vi "Time Profile Logger using LV2.vi"(6 "Command (Log)":T1=enum."Log", 7 "Log Path (Optional)":path, 8 "error in (no error)":errorcluster, 10 "Optional Tags":string[](array[string]), 11 "Primary Tag":string) -> (0 "error out":errorcluster, 2 "Profile Data[][]":string[][](array[string]), 3 "Log Path":path)   [LabVIEW 2016, in "SLL Debug.lvlib"]
doc: "Simple Time Profile Logger with multiple tag inputs. \n\n<b>Important!</b> -The final call to this VI needs to invoke \"Flush and Close\" command to log to file.\n\nDuring logging, the items are just put into a queue. Only during close operation, the data is parsed and logged to file. Supports logging into *.bin, *.csv & *.txt based on the file extension provided to the file name."
uses:
  SLL Debug.lvlib
  _Typedefs/Time Profile Logger Command.ctl
  <vilib>/Utility/file.llb/Write Delimited Spreadsheet (string).vi
  SLL String/SLL String.lvlib
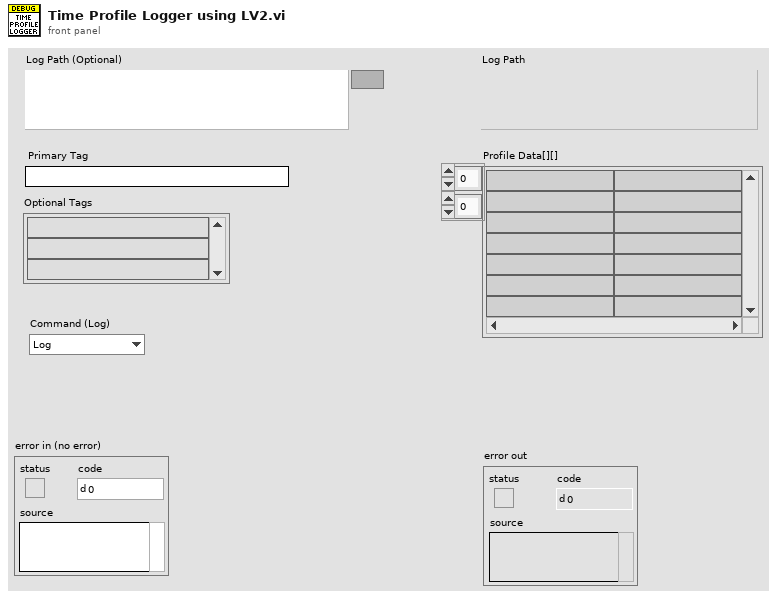
[diagram p1: front panel]
types:
  T1 = typedef "SLL Debug.lvlib/Time Profile Logger Command.ctl" = enum16{"Force Initialize", "Log", "Flush and Close"}
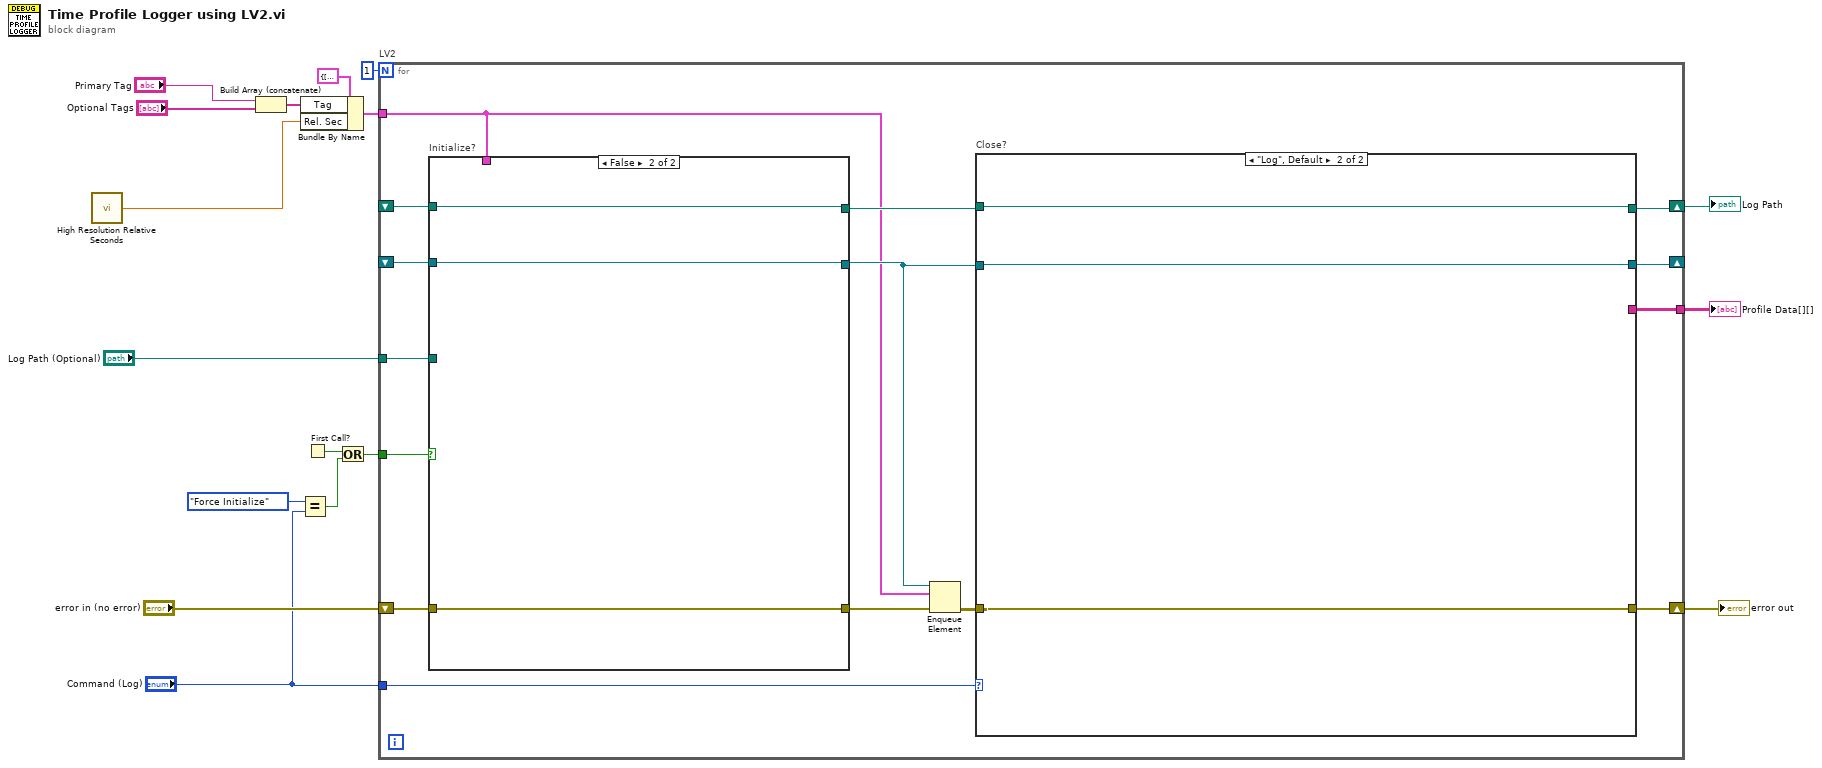
[diagram p0: block diagram]
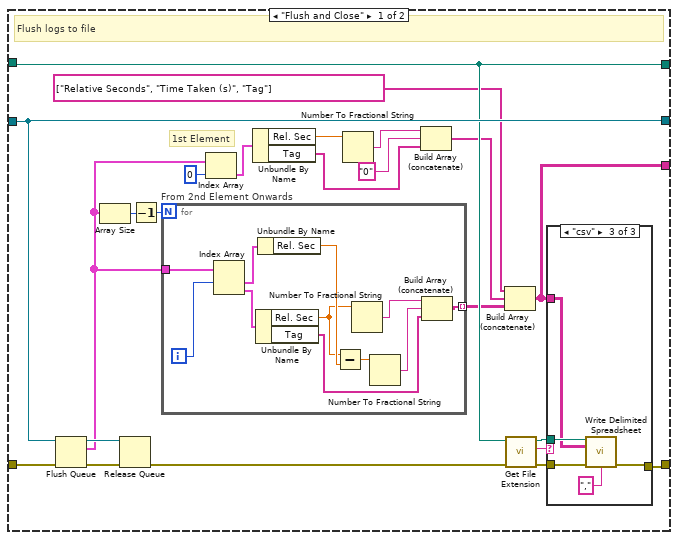
[diagram p2: hidden frame]
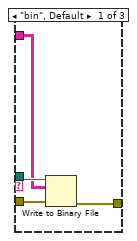
[diagram p3: hidden frame]
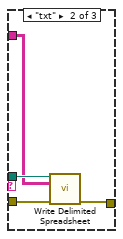
[diagram p4: hidden frame]
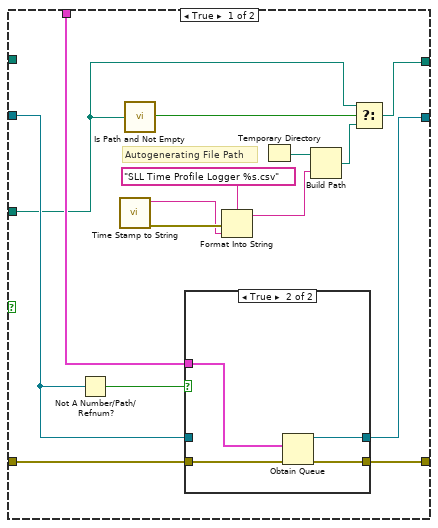
[diagram p5: hidden frame]
diagram:
  n1 = call <vilib>:"High Resolution Relative Seconds.vi"() -> ("relative seconds"=w9:dbl)
  n2 = Build Array (concatenate)("Primary Tag", "Optional Tags") -> (w11:string[])
  n3 = Equal?(x=enum16{"Force Initialize", "Log", "Close"}."Force Initialize", y="Command (Log)") -> (x = y?=w4:bool)
  n4 = Bundle By Name(cluster=cluster{"Tag":string[], "Rel. Sec":dbl} {"Tag"=[], "Rel. Sec"=0.0}, "Tag"=w11, "Rel. Sec"=w9) -> (w10:cluster{"Tag":string[], "Rel. Sec":dbl})
  n5 = First Call?() -> (First Call?: T/F=w5:bool)
  n6 = Or(x=w5, y=w4) -> (x .or. y?=w14:bool)
  n7 = for "LV2" {
    N: 1 -> [_]
    tunnel: w10 -> [w20]
    shift-right: [w21] -> w7
    shift-left: "error in (no error)" -> [w32]
    shift-right: [w23] -> _
    shift-left: _ -> [w31]
    shift-right: [w22] -> w17
    shift-left: _ -> [w30]
    tunnel: w14 -> [w29]
    tunnel: "Command (Log)" -> [w28]
    tunnel: "Log Path (Optional)" -> [w19]
    tunnel: [w18] -> w1
    n8 = case "Initialize?" shown="False" w29 {
      tunnel: w32 -> [w97 w106]
      tunnel: [w96 w106] -> w27
      tunnel: [w95 w105] -> w24
      tunnel: w31 -> [w93 w105]
      tunnel: [w91 w104] -> w25
      tunnel: w30 -> [_ w104]
      tunnel: w20 -> [w90 _]
      tunnel: w19 -> [w89 _]
      frame True {
        # "Autogenerating File Path"
        n9 = Not A Number/Path/Refnum?(number/path/refnum=w93) -> (NaN/Path/Refnum?=w94:bool)
        n10 = call "Time Stamp to String.vi"() -> ("error out"=w88:errorcluster, "Output String"=w86:string)  [unwired: 10 in]
        n11 = call <vilib>:"Is Path and Not Empty.vi"("path"=w89) -> ("Is Path and Not Empty?"=w92:bool)  [unwired: 4 in]
        n12 = case shown="True" w94 {
          tunnel: w97 -> [w98 w103]
          tunnel: [w98 w102] -> w96
          tunnel: [w99 w101] -> w95
          tunnel: w93 -> [w99 _]
          tunnel: w90 -> [_ w100]
          frame False {
          }
          frame True {
            n13 = Obtain Queue(element data type=w100, error in (no error)=w103) -> (queue out=w101:refnum<queue>, error out=w102:errorcluster)  [unwired: 3 in, 1 out]
          }
        }
        n14 = Format Into String(format string="SLL Time Profile Logger %s.csv", error in=w88, w86) -> (resulting string=w84:string)  [unwired: 1 in, 1 out]
        n15 = Temporary Directory() -> (w85:path)
        n16 = Build Path(base path=w85, name or relative path=w84) -> (appended path=w83:path)
        n17 = Select(t=w89, s=w92, f=w83) -> (s? t:f=w91:path)
      }
      frame False {
      }
    }
    n18 = Enqueue Element(queue=w24, element=w20, error in (no error)=w27) -> (error out=w26:errorcluster)  [unwired: 1 in, 2 out]
    n19 = case "Close?" shown="\"Log\", Default" w28 {
      tunnel: w26 -> [w55 w82]
      tunnel: [w46 w82] -> w21
      tunnel: [w53 w81] -> w23
      tunnel: w24 -> [w53 w81]
      tunnel: [w50 w80] -> w22
      tunnel: w25 -> [w50 w80]
      tunnel: [w33 _] -> w18
      frame "Flush and Close" {
        # "1st Element"
        # "Flush logs to file"
        n20 = Flush Queue(queue=w53, error in (no error)=w55) -> (queue out=w52:refnum<queue>, remaining elements=w35:cluster{"Tag":string[], "Rel. Sec":dbl}[], error out=w54:errorcluster)
        n21 = Array Size(array=w35) -> (size(s)=w36:i32)
        n22 = Release Queue(queue=w52, error in (no error)=w54) -> (error out=w51:errorcluster)  [unwired: 1 in, 2 out]
        n23 = Decrement(x=w36) -> (x-1=w37:i32)
        n24 = for "From 2nd Element Onwards" {
          N: w37 -> [_]
          tunnel: w35 -> [w66]
          tunnel: [w60] -> w38 mode=indexing
          i -> [w65]
          n25 = Index Array(array=w66, index #1=w65) -> (element #1=w64:cluster{"Tag":string[], "Rel. Sec":dbl}, element #2=w63:cluster{"Tag":string[], "Rel. Sec":dbl})  [unwired: 1 in]
          n26 = Unbundle By Name(w63) -> ("Rel. Sec"=w58:dbl, "Tag"=w56:string[])
          n27 = Unbundle By Name(w64) -> ("Rel. Sec"=w62:dbl)
          n28 = Subtract(x=w58, y=w62) -> (x-y=w61:dbl)
          n29 = Number To Fractional String(number=w58) -> (F-format string=w57:string)  [unwired: 3 in]
          n30 = Number To Fractional String(number=w61) -> (F-format string=w59:string)  [unwired: 3 in]
          n31 = Build Array (concatenate)(w57, w59, w56) -> (w60:string[])
        }
        n32 = Index Array(array=w35, index=0) -> (element=w40:cluster{"Tag":string[], "Rel. Sec":dbl})
        n33 = Unbundle By Name(w40) -> ("Rel. Sec"=w41:dbl, "Tag"=w34:string[])
        n34 = Number To Fractional String(number=w41) -> (F-format string=w42:string)  [unwired: 3 in]
        n35 = Build Array (concatenate)(w42, "0", w34) -> (w45:string[])
        n36 = Build Array (concatenate)(string[] ["Relative Seconds", "Time Taken (s)", "Tag"], w45, w38) -> (w33:string[][])
        n37 = call <vilib>:"Get File Extension.vi"("error in (no error)"=w51, "file"=w50) -> ("error out"=w48:errorcluster, "lowercase file extension"=w49:string, "dup file"=w47:path)  [unwired: 5 in, 2 out]
        n38 = case shown="\"csv\"" w49 {
          tunnel: w33 -> [w67 w73 w77]
          tunnel: w48 -> [w69 w72 w76]
          tunnel: w47 -> [w70 w74 w79]
          tunnel: [w68 w71 w75] -> w46
          frame "bin", Default {
            n39 = Write to Binary File(file (use dialog)=w70, data=w67, error in=w69) -> (error out=w68:errorcluster)  [unwired: 3 in, 2 out]
          }
          frame "txt" {
            n40 = call-poly <vilib>:"Write Delimited Spreadsheet.vi"("file path (dialog if empty)"=w74, "2D data"=w73, "error in (no error)"=w72) -> ("error out"=w71:errorcluster)  [unwired: 11 in, 1 out]
          }
          frame "csv" {
            n41 = call-poly <vilib>:"Write Delimited Spreadsheet.vi"("file path (dialog if empty)"=w79, "2D data"=w77, "error in (no error)"=w76, "delimiter (\\t)"="," ("delimiter (\\t)")) -> ("error out"=w75:errorcluster)  [unwired: 10 in, 1 out]
          }
        }
      }
      frame "Log", Default {
      }
    }
  }
  "Log Path" <- w17
  "error out" <- w7
  "Profile Data[][]" <- w1
